vi "TDK_SendMsg.vi"(6 "error in (no error)":errorcluster, 7 "CMD":string, 9 "VISA resource name":refnum<visa-resource-name>) -> (0 "error out":errorcluster, 1 "Received Message":string, 3 "VISA resource name":refnum<visa-resource-name>, 4 "Serial Settings:Number of Bytes at Serial Port":u32)   [LabVIEW 2018]
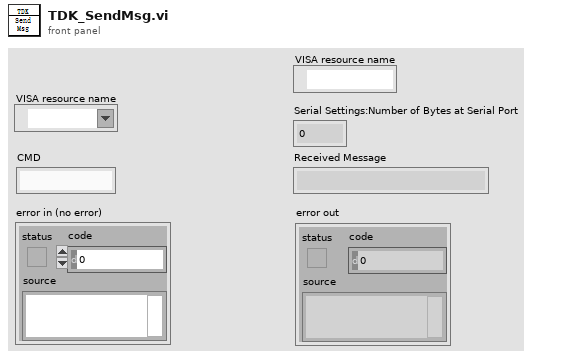
[diagram p1: front panel]
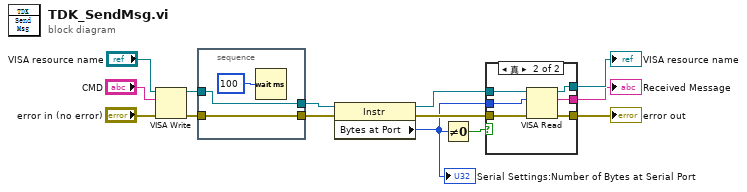
[diagram p0: block diagram]
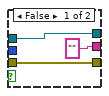
[diagram p2: hidden frame]
diagram:
  n1 = VISA Write(VISA resource name="VISA resource name", write buffer="CMD", error in (no error)="error in (no error)") -> (VISA resource name out=w13:refnum<visa-resource-name>, error out=w14:errorcluster)  [unwired: 1 out]
  n2 = stacked-sequence {
    tunnel: w13 -> [w16]
    tunnel: [w16] -> w6
    tunnel: w14 -> [w15]
    tunnel: [w15] -> w5
    frame #0 {
      n3 = Wait (ms)(milliseconds to wait=u32 100) -> ()  [unwired: 1 out]
    }
  }
  n4 = property class="Instr"(reference=w6, error in=w5) -> (reference out=w4:refnum<visa-resource-name>, error out=w3:errorcluster, "Bytes at Port"=w1:u32)
  "Serial Settings:Number of Bytes at Serial Port" <- w1
  n5 = Not Equal To 0?(x=w1) -> (x != 0?=w2:bool)
  n6 = case shown="真" w2 {
    tunnel: [w18 w26] -> w12
    tunnel: [w19 w25] -> w11
    tunnel: ["" ("read buffer") w24] -> w9
    tunnel: w4 -> [w19 w23]
    tunnel: w3 -> [w18 w22]
    tunnel: w1 -> [_ w21]
    frame False {
    }
    frame True {
      n7 = VISA Read(VISA resource name=w23, byte count=w21, error in (no error)=w22) -> (VISA resource name out=w25:refnum<visa-resource-name>, read buffer=w24:string, error out=w26:errorcluster)  [unwired: 1 out]
    }
  }
  "VISA resource name" <- w11
  "error out" <- w12
  "Received Message" <- w9
